vi "MFRWV Mass Flow Rate of Water Vapor in Air in Humid Air (Kg to S).vi"(1 "Gas Presure":dbl[unit]=80000.0 min=80000.0 max=120000.0, 2 "Tceg":dbl[unit], 3 "MFRHA\nMass Flow Rate of Humid Air (Kg/s)":dbl[unit], 4 "RH":dbl) -> (0 "MFRWV":dbl[unit])   [LabVIEW 2018]
panel:
  out "MFRWV\nMass Flow Rate of Water Vapor in\nAir in Humid Air\nMFRWV=MFRHA-MFRDA;":dbl[unit](knob) scale=0.0..10.0
  out "Temprature Of Input Air\nCentigrade Degree":dbl[unit](slide) scale=0.0..100.0
  out "Humidity of Input Air":dbl(knob) scale=0.0..100.0
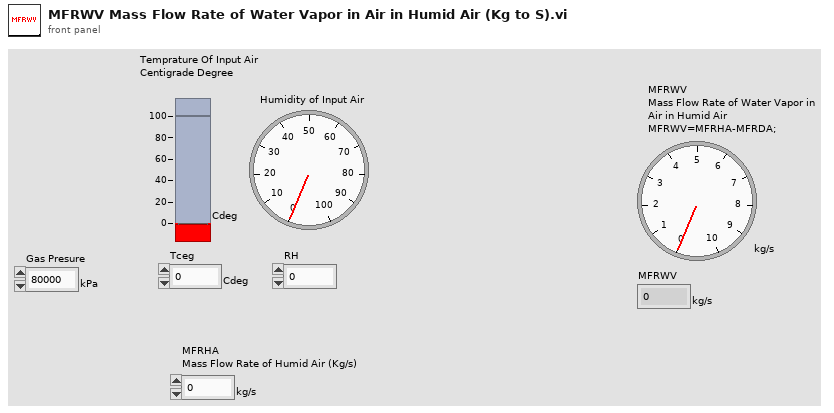
[diagram p1: front panel]
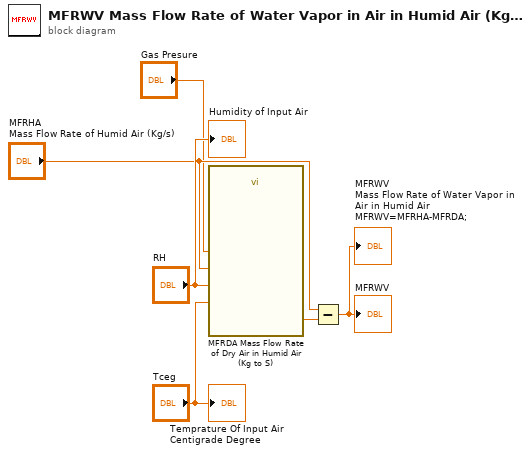
[diagram p0: block diagram]
diagram:
  n1 = call "MFRDA Mass Flow Rate of Dry Air in Humid Air (Kg to S).vi"("Gas Presure"="Gas Presure", "Tceg"="Tceg", "MFRHA\nMass Flow Rate of Humid Air (Kg/s)"="MFRHA\nMass Flow Rate of Humid Air (Kg/s)", "RH"="RH") -> ("MFRDA"=w5:dbl[unit])
  n2 = Subtract(x="MFRHA\nMass Flow Rate of Humid Air (Kg/s)", y=w5) -> (x-y=→"MFRWV\nMass Flow Rate of Water Vapor in\nAir in Humid Air\nMFRWV=MFRHA-MFRDA;" →"MFRWV":dbl[unit])
  "Humidity of Input Air" <- "RH"
  "Temprature Of Input Air\nCentigrade Degree" <- "Tceg"
